vi "网页.vi"() -> ()   [LabVIEW 2018]
panel:
  in  "WebBrowser":refnum<k7>(container) caption="网页浏览器"
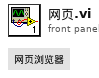
[diagram p1: front panel]
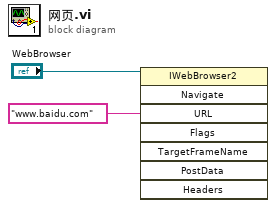
[diagram p0: block diagram]
diagram:
  n1 = invoke class="IWebBrowser2" method="Navigate"(reference="WebBrowser", "URL"="www.baidu.com") -> ()  [unwired: 6 in, 8 out]
